vi "AddMessage.vi"(4 "add newline":bool, 5 "message":string, 6 "error in":errorcluster, 9 "MessageBox in":refnum<class "MessageBox.lvclass">) -> (0 "error out":errorcluster, 3 "MessageBox out":refnum<class "MessageBox.lvclass">)   [LabVIEW 2014, in "MessageBox.lvclass"]
uses:
  MessageBox.lvclass
  MessageBox.lvclass/MessageBox.ctl
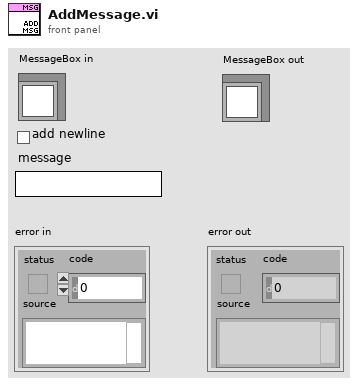
[diagram p1: front panel]
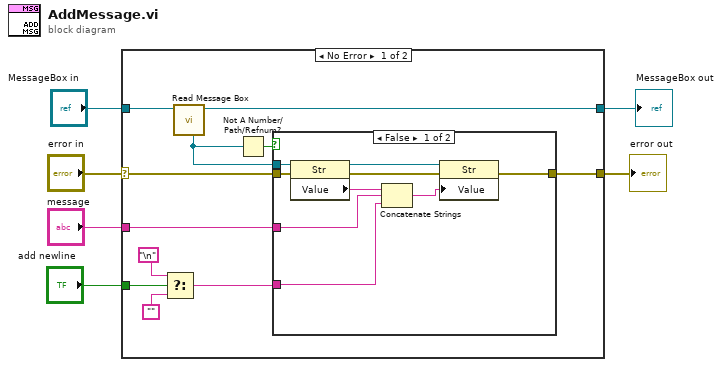
[diagram p0: block diagram]
diagram:
  n1 = case shown="No Error" "error in" {
    selector: "error in" -> [w10 w29]
    tunnel: [w9 w29] -> w5
    tunnel: [w16 w28] -> w1
    tunnel: "MessageBox in" -> [w17 w28]
    tunnel: "message" -> [w15 _]
    tunnel: "add newline" -> [w14 _]
    frame No Error {
      n2 = Select(t="\n", s=w14, f="") -> (s? t:f=w11:string)
      n3 = call "Read Message Box.vi"("MessageBox in"=w17) -> ("MessageBox out"=w16:refnum<class "MessageBox.lvclass">, "Message Box"=w7:refnum<vi>)  [unwired: 7 in]
      n4 = Not A Number/Path/Refnum?(number/path/refnum=w7) -> (NaN/Path/Refnum?=w8:bool)
      n5 = case shown="False" w8 {
        tunnel: w7 -> [w26 _]
        tunnel: w15 -> [w24 _]
        tunnel: w11 -> [w23 _]
        tunnel: w10 -> [w19 w27]
        tunnel: [w18 w27] -> w9
        frame False {
          n6 = property class="Str"(reference=w26, error in=w19) -> (reference out=w21:refnum<vi>, error out=w22:errorcluster, "Value"=w25:string)
          n7 = Concatenate Strings(w25, w24, w23) -> (w20:string)
          n8 = property class="Str"(reference=w21, error in=w22, "Value"=w20) -> (error out=w18:errorcluster)  [unwired: 1 out]
        }
        frame True {
        }
      }
    }
    frame Error {
    }
  }
  "error out" <- w5
  "MessageBox out" <- w1
